vi "cal_main_format_const_pos.vi"(5 "Main Node BD Position":cluster{"Left":i32, "Top":i32}, 11 "error in (no error)":errorcluster) -> (6 "Constant Position":cluster{"Left":i32, "Top":i32}, 15 "error out":errorcluster)   [LabVIEW 2018]
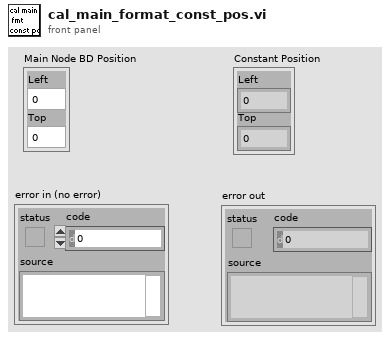
[diagram p1: front panel]
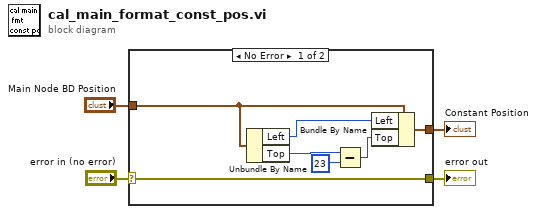
[diagram p0: block diagram]
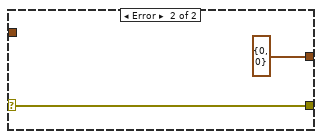
[diagram p2: hidden frame]
diagram:
  n1 = case shown="No Error" "error in (no error)" {
    selector: "error in (no error)" -> [w6 w12]
    tunnel: "Main Node BD Position" -> [w11 _]
    tunnel: [w10 cluster{"Left":i32, "Top":i32} {"Left"=0, "Top"=0} ("Main Node BD Position")] -> w3
    tunnel: [w6 w12] -> w1
    frame No Error {
      n2 = Unbundle By Name(w11) -> ("Left"=w5:i32, "Top"=w7:i32)
      n3 = Subtract(x=w7, y=23) -> (x-y=w9:i32)
      n4 = Bundle By Name(cluster=w11, "Left"=w5, "Top"=w9) -> (w10:cluster{"Left":i32, "Top":i32})
    }
    frame Error {
    }
  }
  "Constant Position" <- w3
  "error out" <- w1
